vi "Make Box on Graph.vi"(6 "Theta":dbl, 8 "Y2":dbl, 9 "Y1":dbl, 10 "X2":dbl, 11 "X1":dbl) -> (3 "Output Graph":cluster{dbl[], dbl[]})   [LabVIEW 2019]
uses:
  <vilib>/Analysis/coordinate.llb/2D Cartesian Coordinate Rotation (Array).vi
  <vilib>/Analysis/NI_AALPro.lvlib
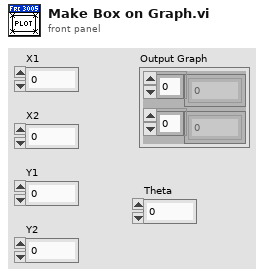
[diagram p1: front panel]
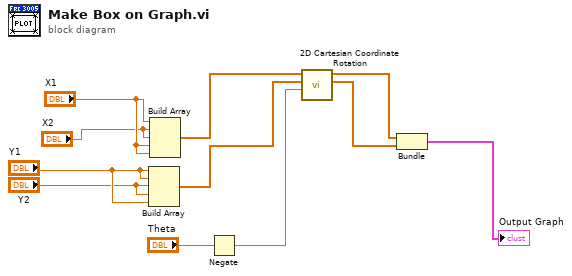
[diagram p0: block diagram]
diagram:
  n1 = Build Array("Y1", "Y1", "Y2", "Y2", "Y1") -> (w4:dbl[])
  n2 = Build Array("X1", "X2", "X2", "X1", "X1") -> (w6:dbl[])
  n3 = Negate(x="Theta") -> (-x=w1:dbl)
  n4 = call-poly <vilib>:"2D Cartesian Coordinate Rotation.vi"("theta"=w1, "Y"=w4, "X"=w6) -> ("Y Out"=w3:dbl[], "X Out"=w5:dbl[])  [unwired: 6 in, 1 out]
  n5 = Bundle("X Out"=w5, "Y Out"=w3) -> (→"Output Graph":cluster{"X Out":dbl[], "Y Out":dbl[]})  [unwired: 1 in]
